vi "Set_SG394_Mode.vi"(4 "Modulation type":u16(ring) items=["AM/ASK"=0, "FM/FSK"=1, "PM/PSK"=2, "Sweep"=3, "Pulse"=4, "Blank"=5, "QAM"=7, "CPM"=8, "VSB"=9], 5 "Modulation":bool=TRUE, 6 "N type Amplitude (-110 to 0 dBm)":dbl min=-110.0 max=0.0, 7 "BNC Amplitude (-47 to 0 dBm)":dbl min=-110.0 max=0.0, 8 "error in (no error)":errorcluster, 9 "N type output":bool=TRUE, 10 "BNC output":bool=TRUE, 11 "VISA resource name":refnum<visa-resource-name>="GPIB0::27::INSTR") -> (0 "error out":errorcluster, 3 "VISA resource name out":refnum<visa-resource-name>)   [LabVIEW 2015]
uses:
  Libraries/Stanford Research SG39x Series/Stanford Research SG39x Series.lvlib
panel:
  # "IQ modulation ON: QAM\nIQ modulation OFF: Pulse"
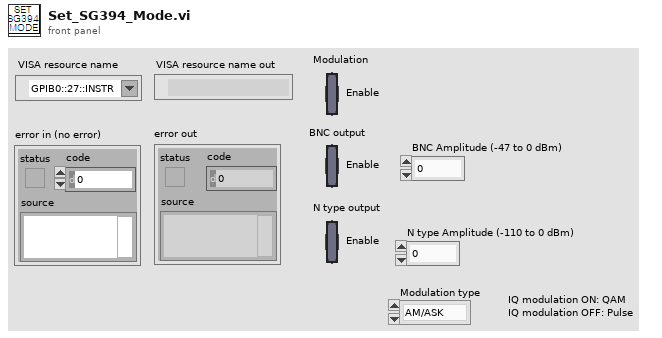
[diagram p1: front panel]
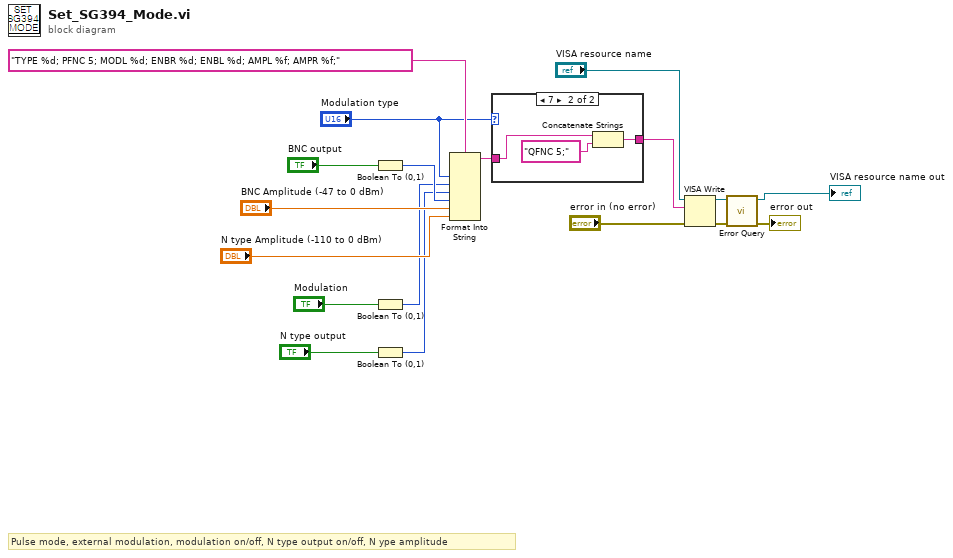
[diagram p0: block diagram]
diagram:
  # "Pulse mode, external modulation, modulation on/off, N type output on/off, N ype amplitude"
  n1 = Boolean To (0,1)(Boolean="BNC output") -> (0, 1=w7:i16)
  n2 = Boolean To (0,1)(Boolean="Modulation") -> (0, 1=w5:i16)
  n3 = Boolean To (0,1)(Boolean="N type output") -> (0, 1=w6:i16)
  n4 = Format Into String(format string="TYPE %d; PFNC 5; MODL %d; ENBR %d; ENBL %d; AMPL %f; AMPR %f;", "Modulation type", w5, w6, w7, "BNC Amplitude (-47 to 0 dBm)", "N type Amplitude (-110 to 0 dBm)") -> (resulting string=w2:string)  [unwired: 2 in, 1 out]
  n5 = case shown="7" "Modulation type" {
    tunnel: w2 -> [w19 w22]
    tunnel: [w19 w20] -> w1
    frame 0, Default {
    }
    frame 7 {
      n6 = Concatenate Strings(w22, "QFNC 5;") -> (w20:string)
    }
  }
  n7 = VISA Write(VISA resource name="VISA resource name", write buffer=w1, error in (no error)="error in (no error)") -> (VISA resource name out=w17:refnum<visa-resource-name>, error out=w16:errorcluster)  [unwired: 1 out]
  n8 = call "Error Query.vi"("error in (no error)"=w16, "VISA resource name"=w17) -> ("error out"=→"error out":errorcluster, "VISA resource name out"=→"VISA resource name out":refnum<visa-resource-name>)  [unwired: 6 in, 2 out]
